vi "Pockels Cal-Source-Default power meter cal.vi"() -> (3 "Default power meter cal":string[][](array[string]))   [LabVIEW 2017]
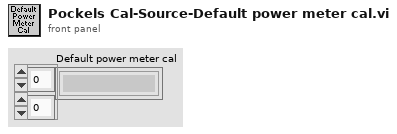
[diagram p1: front panel]
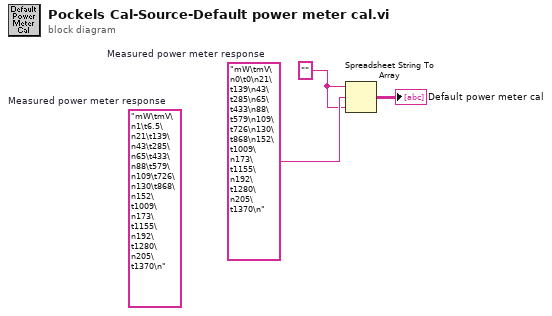
[diagram p0: block diagram]
diagram:
  (unwired) "mW\tmV\n1\t6.5\n21\t139\n43\t285\n65\t433\n88\t579\n109\t726\n130\t868\n152\t1009\n173\t1155\n192\t1280\n205\t1370\n"  # Measured power meter response
  w3 = "mW\tmV\n0\t0\n21\t139\n43\t285\n65\t433\n88\t579\n109\t726\n130\t868\n152\t1009\n173\t1155\n192\t1280\n205\t1370\n"  # Measured power meter response
  w1 = "" ("format string")
  n1 = Spreadsheet String To Array(format string=w1, spreadsheet string=w3, array type (2D Dbl)=w1) -> (array=→"Default power meter cal":string[][])  [unwired: 1 in]
